vi "子VI-查看某框.vi"(0 "输入框号（默认值0为整张图）":dbl format="%#_13g", 1 "框组":T3(array[cluster]), 2 "判定为筋条的长宽比阈值":i32, 3 "临界Z值":i32, 4 "缺陷灰度阈值":dbl caption="值", 5 "临界面积百分比值":dbl, 6 "计入缺陷的面积阈值":i32, 7 "计入缺陷的Z值阈值":i32 caption="值", 8 "?":T2(plugin-control), 9 "部位信息":string[](array[string])=["", "34.500000", "32.500000", "1121", "34", "54.955926", "分层类", "不合格", ""], 10 "图像Y向分辨率（mm/像素）":dbl, 11 "图像X向分辨率（mm/像素）":dbl) -> (27 "全部检测结果":string[][](table))   [LabVIEW 2018]
uses:
  <vilib>/vision/NI_Vision_Development_Module.lvlib
panel:
  out "测量结果":dbl[][](array[numeric])
  out "中心Y":dbl
  out "中心X":dbl
  in  "返回主界面":bool caption="辅助定性分析"
  in  "Tab Control":T1
  out "?":T2(plugin-control)
  out "Threshold Image":T2(plugin-control)
  out "分层缺陷个数":i32
  out "合格？ 弥散类":string="fencengThreshold"
  out "合格？分层类":string="fencengThreshold"
  out "?":string
  out "面积 (pixels)":i32
  in  "格式字符串 2":string="%f"
  in  "分隔符（'\\'代码显示）":string="\t"
  out "分层测量结果":dbl[][](array[numeric])
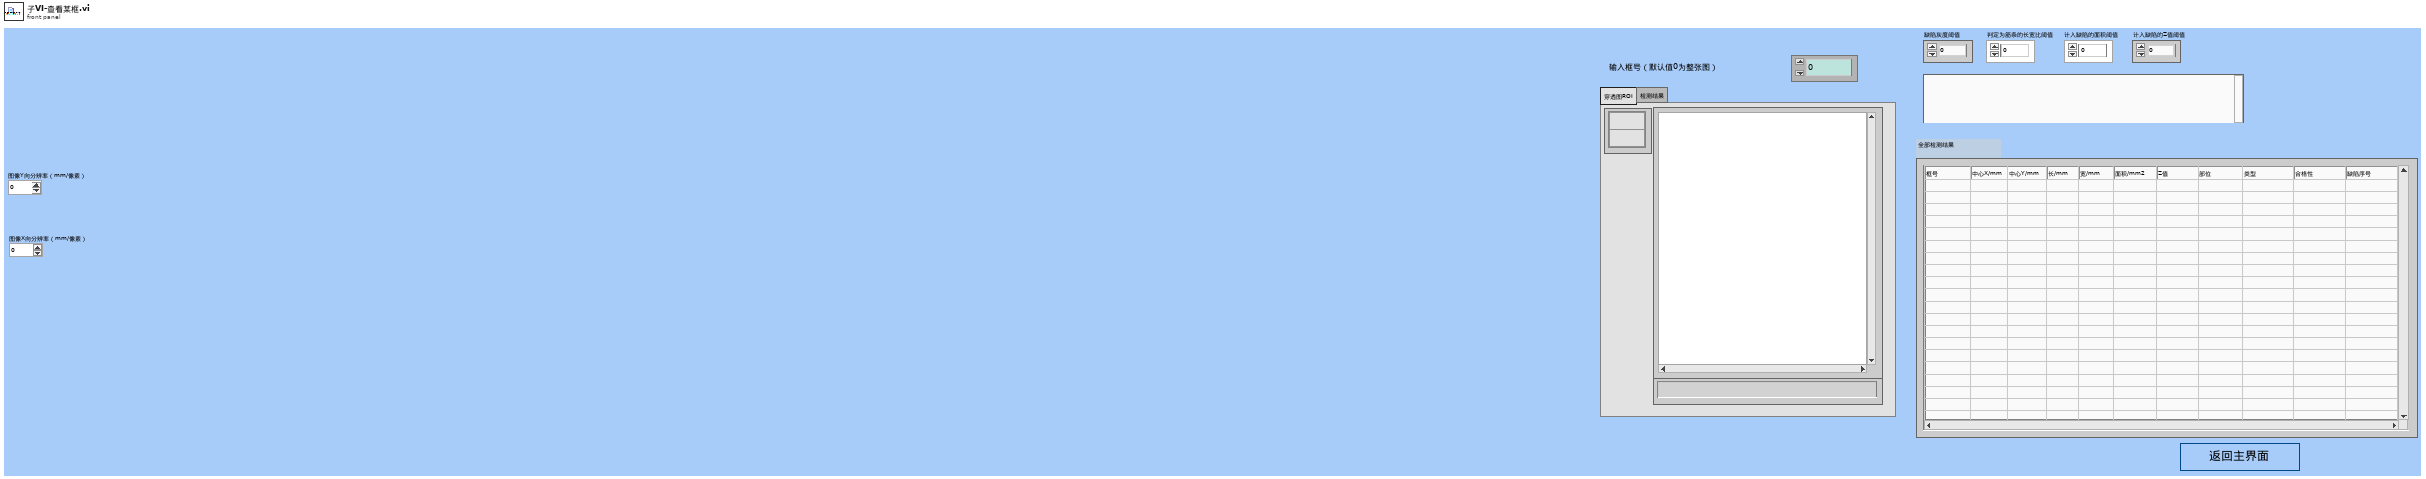
[diagram p1: front panel]
types:
  T1 = typedef "控件2.ctl" = enum32{"穿透图ROI", "检测结果"}
  T2 = typedef "IMAQ Image.ctl" = refnum<image>
  T3 = cluster{"Global Rectangle":i32[], "Contours":cluster{"Contour Type":u32, "ROI Type":u32, "Points":i32[]}[]}[]
  T4 = cluster{"Desired Font (Application)":enum16{"User-specified Font", "Application Font", "System Font", "Dialog Font"}, "[User-specified Font]":cluster{"Font Name":string, "Size":i16, "Strikeout?":bool, "Italic?":bool, "Underline?":bool, "Outline?":bool, "Shadow?":bool, "Bold?":bool, "Rotation Angle":dbl}, "Horizontal Alignment":i16, "Vertical Alignment":i16}
  T5 = cluster{"Zoom Tool":bool, "Selection Tool":bool, "Pan Tool":bool, "Point Tool":bool, "Line Tool":bool, "Rectangle Tool":bool, "Rotated Rectangle Tool":bool, "Polyline Tool":bool, "Polygon Tool":bool, "Freehand Tool":bool, "Closed Freehand Tool":bool, "Ellipse Tool":bool, "Annulus Tool":bool}
  T6 = typedef "Image Type" = u32
  T7 = cluster{"Global Rectangle":i32[], "Contours":cluster{"Contour Type":u32, "ROI Type":u32, "Points":i32[]}[]}
  T8 = cluster{"histogram":u32[], "Minimal Value":sgl, "Maximal Value":sgl, "Starting Value":sgl, "Interval Width":sgl, "Mean Value":sgl, "Standard  Variation":sgl, "Area (pixels)":i32}
  T9 = typedef "Particle Parameters" = i32
  T10 = cluster{"Area":dbl, "Number of Holes":dbl, "Bounding Rect":cluster{"Left":dbl, "Top":dbl, "Right":dbl, "Bottom":dbl}, "Center of Mass":cluster{"X":dbl, "Y":dbl}, "Orientation":dbl, "Dimensions":cluster{"Width":dbl, "Height":dbl}}[]
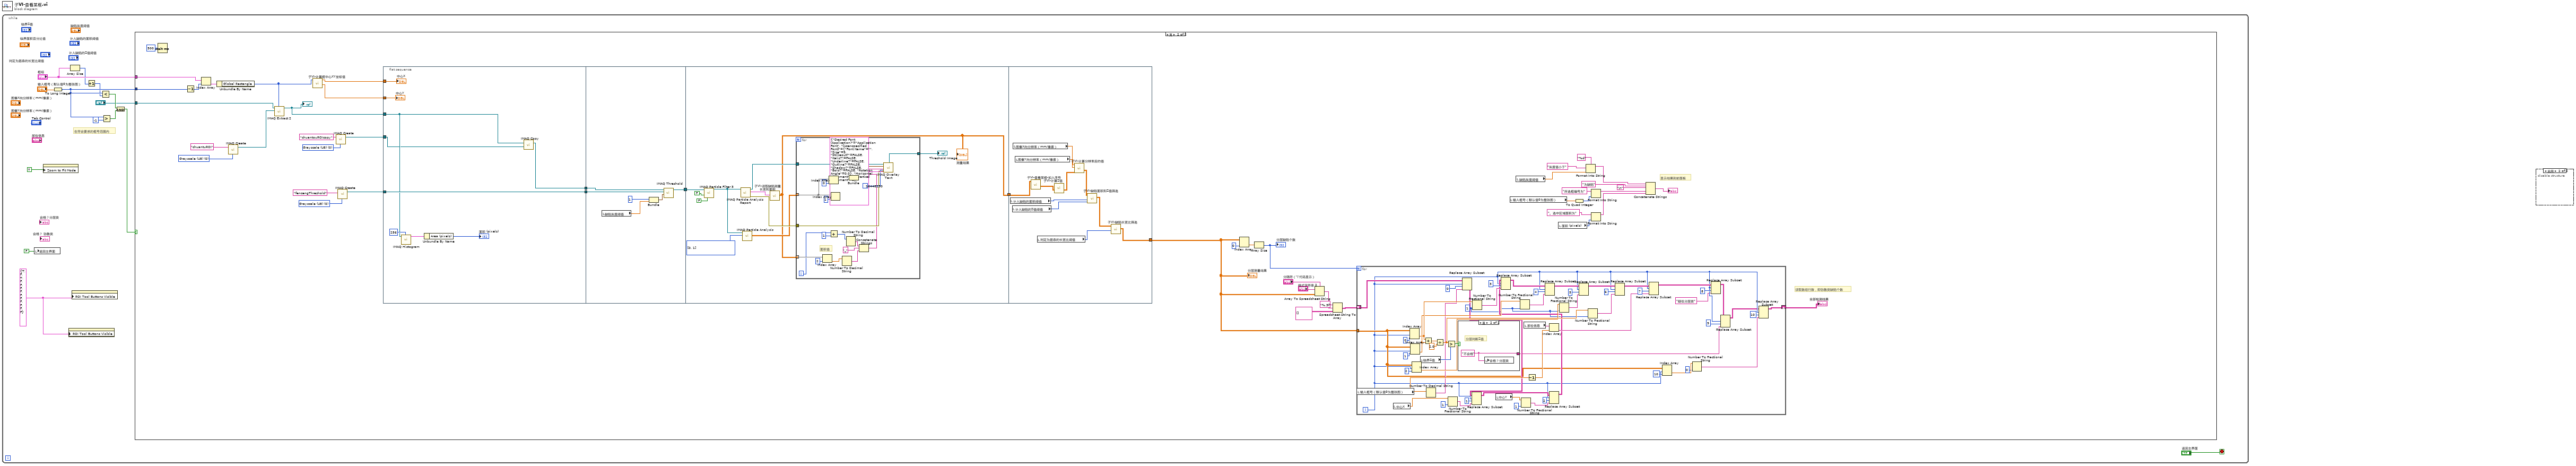
[diagram p0: block diagram]
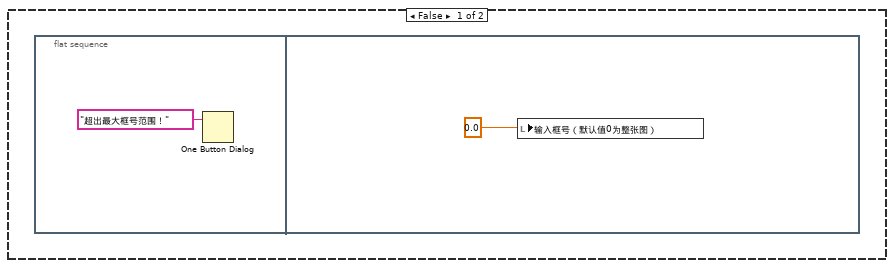
[diagram p2: hidden frame]
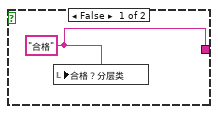
[diagram p3: hidden frame]
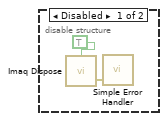
[diagram p4: hidden frame]
diagram:
  n1 = while {
    stop <- "返回主界面" stop-if-true
    w4 = T5 {"Zoom Tool"=TRUE, "Selection Tool"=FALSE, "Pan Tool"=TRUE, "Point Tool"=FALSE, "Line Tool"=FALSE, "Rectangle Tool"=FALSE, "Rotated Rectangle Tool"=FALSE, "Polyline Tool"=FALSE, "Polygon Tool"=FALSE, "Freehand Tool"=FALSE, "Closed Freehand Tool"=FALSE, "Ellipse Tool"=FALSE, "Annulus Tool"=FALSE} ("ROI Tool Buttons Visible:All Elements")
    # "在符合要求的框号范围内"
    n2 = local write "返回主界面"(FALSE ("stop")) -> ()
    n3 = property class="ImageControl"("Zoom to Fit Mode"=TRUE) -> ()  [unwired: 2 in, 2 out]
    n4 = To Long Integer(number="输入框号（默认值0为整张图）") -> (32bit integer=w6:i32)
    n5 = property class="ImageControl"("ROI Tool Buttons Visible"=w4) -> ()  [unwired: 2 in, 2 out]
    n6 = Array Size(array="框组") -> (size(s)=w3:i32)
    n7 = property class="ImageControl"("ROI Tool Buttons Visible"=w4) -> ()  [unwired: 2 in, 2 out]
    n8 = Increment(x=w3) -> (x+1=w2:i32)
    n9 = Less?(x=w6, y=w2) -> (x < y?=w8:bool)
    n10 = Greater?(x=w6, y=-1) -> (0:w7:bool)
    n11 = And(x=w8, y=w7) -> (x .and. y?=w9:bool)
    n12 = case shown="真" w9 {
      tunnel: "框组" -> [_ w29]
      tunnel: w6 -> [_ w28]
      tunnel: "?" -> [_ w20]
      frame False {
        n13 = flat-sequence {
          frame #0 {
            n14 = One Button Dialog(message="超出最大框号范围！" ("消息")) -> ()  [unwired: 1 in, 1 out]
          }
          frame #1 {
            n15 = local write "输入框号（默认值0为整张图）"(0.0 ("框号")) -> ()
          }
        }
      }
      frame True {
        w43 = T6 0 items=["Grayscale (U8)", "Grayscale (I16)", "Grayscale (SGL)", "Complex (CSG)", "RGB (U32)", "HSL (U32)", "RGB (U64)", "Grayscale (U16)"] ("Image Type")
        w55 = T6 0 items=["Grayscale (U8)", "Grayscale (I16)", "Grayscale (SGL)", "Complex (CSG)", "RGB (U32)", "HSL (U32)", "RGB (U64)", "Grayscale (U16)"] ("Image Type")
        w57 = T6 0 items=["Grayscale (U8)", "Grayscale (I16)", "Grayscale (SGL)", "Complex (CSG)", "RGB (U32)", "HSL (U32)", "RGB (U64)", "Grayscale (U16)"] ("Image Type")
        # "显示结果到前面板"
        # "读取数组行数，即弥散类缺陷个数"
        n16 = Wait (ms)(milliseconds to wait=u32 500 ("等待时间（毫秒）")) -> ()  [unwired: 1 out]
        n17 = Decrement(x=w28) -> (x-1=w60:i32)
        n18 = Index Array(array=w29, index=w60) -> (element=w61:T7)
        n19 = Unbundle By Name(w61) -> ("Global Rectangle"=w25:i32[])
        n20 = call "IMAQ Create"("Image Name"="chuantuROI", "Image Type"=w57) -> ("New Image"=w56:T2)  [unwired: 3 in, 1 out]
        n21 = call "IMAQ Extract 2"("Optional Rectangle"=w25, "Image Dst"=w56, "Image Src"=w20) -> ("Image Dst Out"=w19:T2)  [unwired: 7 in, 1 out]
        "?" <- w19
        n22 = call "子VI-计算框中心XY坐标值.vi"("Global Rectangle"=w25) -> ("中心Y"=w23:dbl, "中心X"=w22:dbl)  [unwired: 9 in]
        n23 = call "IMAQ Create"("Image Name"="chuantouROIcopy", "Image Type"=w43) -> ("New Image"=w45:T2)  [unwired: 3 in, 1 out]
        n24 = call "IMAQ Create"("Image Name"="fencengThreshold", "Image Type"=w55) -> ("New Image"=w52:T2)  [unwired: 3 in, 1 out]
        n25 = flat-sequence {
          tunnel: [w133] -> w64
          tunnel: [w128] -> w63
          tunnel: w52 -> [w133]
          tunnel: w19 -> [w129]
          tunnel: w45 -> [w127]
          tunnel: w23 -> [w126]
          tunnel: w22 -> [w125]
          tunnel: w64 -> [w139]
          tunnel: [w134] -> w62
          tunnel: w63 -> [w138]
          tunnel: w62 -> [w147]
          tunnel: [w140] -> w18
          tunnel: [w178] -> w21
          tunnel: w18 -> [w177]
          frame #0 {
            n26 = call "IMAQ Histogram"("Number of Classes"=256, "Image"=w129) -> ("Histogram Report"=w131:T8)  [unwired: 8 in, 1 out]
            n27 = Unbundle By Name(w131) -> ("Area (pixels)"=→"面积 (pixels)":i32)
            n28 = call "IMAQ Copy"("Image Dst"=w127, "Image Src"=w129) -> ("Image Dst Out"=w128:T2)  [unwired: 4 in, 1 out]
            "中心Y" <- w126
            "中心X" <- w125
          }
          frame #1 {
            n29 = local read "缺陷灰度阈值"() -> (w135:dbl)
            n30 = Bundle(1, "缺陷灰度阈值"=w135) -> (w137:cluster{i32, "缺陷灰度阈值":dbl})  [unwired: 1 in]
            n31 = call "IMAQ Threshold"("Range"=w137, "Image Dst"=w139, "Image Src"=w138) -> ("Image Dst Out"=w134:T2)  [unwired: 3 in, 5 out]
          }
          frame #2 {
            w141 = T9[] [0, 1] items=["Center of Mass X", "Center of Mass Y", "First Pixel X", "First Pixel Y", "Bounding Rect Left", "Bounding Rect Top", "Bounding Rect Right", "Bounding Rect Bottom", "Max Feret Diameter Start X", "Max Feret Diameter Start Y", "Max Feret Diameter End X", "Max Feret Diameter End Y", "Max Horiz. Segment Length Left", "Max Horiz. Segment Length Right", "Max Horiz. Segment Length Row", "-", "Bounding Rect Width", "Bounding Rect Height", "Bounding Rect Diagonal", "Perimeter", "Convex Hull Perimeter", "Holes' Perimeter", "Max Feret Diameter", "Equivalent Ellipse Major Axis", "Equivalent Ellipse Minor Axis", "Equivalent Ellipse Minor Axis (Feret)", "Equivalent Rect Long Side", "Equivalent Rect Short Side", "Equivalent Rect Diagonal", "Equivalent Rect Short Side (Feret)", "Average Horiz. Segment Length", "Average Vert. Segment Length", "Hydraulic Radius", "Waddel Disk Diameter", "-", "Area", "Holes' Area", "Particle & Holes' Area", "Convex Hull Area", "Image Area", "-", "Number of Holes", "Number of Horiz. Segments", "Number of Vert. Segments", "-", "Orientation", "Max Feret Diameter Orientation", "-", "% Area/Image Area", "% Area/(Particle & Holes' Area)", "Ratio of Equivalent Ellipse Axes", "Ratio of Equivalent Rect Sides", "-", "Elongation Factor", "Compactness Factor", "Heywood Circularity Factor", "Type Factor", "-", "Sum X", "Sum Y", "Sum XX", "Sum XY", "Sum YY", "Sum XXX", "Sum XXY", "Sum XYY", "Sum YYY", "-", "Moment of Inertia XX", "Moment of Inertia XY", "Moment of Inertia YY", "Moment of Inertia XXX", "Moment of Inertia XXY", "Moment of Inertia XYY", "Moment of Inertia YYY", "Norm. Moment of Inertia XX", "Norm. Moment of Inertia XY", "Norm. Moment of Inertia YY", "Norm. Moment of Inertia XXX", "Norm. Moment of Inertia XXY", "Norm. Moment of Inertia XYY", "Norm. Moment of Inertia YYY", "Hu Moment 1", "Hu Moment 2", "Hu Moment 3", "Hu Moment 4", "Hu Moment 5", "Hu Moment 6", "Hu Moment 7"] ("Pixel Measurements")
            n32 = call "IMAQ Particle Filter 3"("Image Src"=w147, "Keep/Remove Particles (F)"=FALSE, "Reject Border? (F)"=FALSE) -> ("Image Dst Out"=w143:T2)  [unwired: 10 in, 2 out]
            n33 = call "IMAQ Particle Analysis Report"("Image"=w143) -> ("error out"=w144:errorcluster, "Particle Reports (Pixels)"=w148:T10, "Image Out (duplicate)"=w145:T2)  [unwired: 5 in, 3 out]
            n34 = call "IMAQ Particle Analysis"("Pixel Measurements"=w141, "Image"=w143) -> ("Particle Measurements (Pixels)"=w142:dbl[][])  [unwired: 4 in, 5 out]
            n35 = call "子VI-读取缺陷测量长宽和面积.vi"("Particle Reports (Pixels)"=w148) -> ("测量结果"=w140:dbl[][])  [unwired: 10 in]
            "测量结果" <- w140
            n36 = for {
              tunnel: [w163] -> w146
              tunnel: w145 -> [w171]
              tunnel: w142 -> [w168] mode=indexing
              tunnel: w144 -> [w162]
              tunnel: w140 -> [w158] mode=indexing
              i -> [w153]
              # "面积值"
              n37 = Index Array(array=w158, index=2 ("索引")) -> (element=w166:dbl)
              n38 = Index Array(array=w168, index=0 ("索引")) -> (element=w161:dbl)
              n39 = Add(x=w153, y=1) -> (x+y=w151:i32)
              n40 = Index Array(array=w168, index=1 ("索引")) -> (element=w160:dbl)
              n41 = Number To Decimal String(number=w166) -> (decimal integer string=w155:string)  [unwired: 1 in]
              n42 = Number To Decimal String(number=w151) -> (decimal integer string=w157:string)  [unwired: 1 in]
              n43 = Bundle("Numeric"=w161, "Numeric"=w160) -> (w159:cluster{"Numeric":dbl, "Numeric":dbl})  [unwired: 1 in]
              n44 = Concatenate Strings(w157, "_" ("字符串"), w155) -> (w156:string)
              n45 = call "IMAQ Overlay Text"("Text Color (black)"=u32 16448250, "Font, Size & Style"=T4 {"Desired Font (Application)"=enum."Application Font", "[User-specified Font]"={"Font Name"="", "Size"=9, "Strikeout?"=FALSE, "Italic?"=FALSE, "Underline?"=FALSE, "Outline?"=FALSE, "Shadow?"=FALSE, "Bold?"=FALSE, "Rotation Angle"=0.0}, "Horizontal Alignment"=0, "Vertical Alignment"=0}, "error in (no error)"=w162, "String"=w156, "Origin"=w159, "Image"=w171) -> ("Image Out"=w163:T2)  [unwired: 4 in, 1 out]
            }
            "Threshold Image" <- w146
          }
          frame #3 {
            n46 = local read "计入缺陷的面积阈值"() -> (w179:i32)
            n47 = local read "计入缺陷的Z值阈值"() -> (w176:i32)
            n48 = local read "图像X向分辨率（mm/像素）"() -> (w181:dbl)
            n49 = local read "图像Y向分辨率（mm/像素）"() -> (w182:dbl)
            n50 = call "子VI-查看某框-加入序号.vi"("测量结果"=w177) -> ("测量结果 3"=w175:dbl[][])  [unwired: 9 in]
            n51 = local read "判定为筋条的长宽比阈值"() -> (w180:i32)
            n52 = call "子VI-计算Z值.vi"("分层测量结果"=w175) -> ("初始化的数组"=w174:dbl[][])  [unwired: 9 in]
            n53 = call "子VI-计算分辨率后的值.vi"("测量结果"=w174, "图像X向分辨率（mm/像素）"=w181, "图像Y向分辨率（mm/像素）"=w182) -> ("初始化的数组"=w173:dbl[][])  [unwired: 7 in]
            n54 = call "子VI-缺陷面积和Z值筛选.vi"("计入缺陷的Z值阈值"=w176, "计入分层缺陷的面积阈值"=w179, "分层测量结果"=w173) -> ("初始化的数组"=w172:dbl[][])  [unwired: 7 in, 1 out]
            n55 = call "子VI-缺陷长宽比筛选.vi"("判定为筋条的长宽比阈值"=w180, "分层测量结果"=w172) -> ("初始化的数组"=w178:dbl[][])  [unwired: 9 in]
          }
        }
        n56 = Index Array(array=w21, index (col)=0 ("禁用的索引 (列)")) -> (element=w54:dbl[])  [unwired: 1 in]
        n57 = Array Size(array=w54) -> (size(s)=w51:i32)
        "分层缺陷个数" <- w51
        n58 = Array To Spreadsheet String(delimiter (Tab)="分隔符（'\\'代码显示）", array=w21, 3:"格式字符串 2") -> (spreadsheet string=w48:string)
        n59 = Spreadsheet String To Array(format string="%.3f" ("格式字符串"), spreadsheet string=w48, array type (2D Dbl)=string[][] [] ("Array")) -> (array=w46:string[][])  [unwired: 1 in]
        n60 = for {
          N: w51 -> [_]
          tunnel: w21 -> [w74]
          shift-right: [w69] -> w17
          shift-left: w46 -> [w106]
          i -> [w71]
          w79 = i16 1 ("精度(6)")
          n61 = local read "输入框号（默认值0为整张图）"() -> (w113:dbl)
          n62 = local read "中心X"() -> (w90:dbl)
          n63 = Index Array(array=w74, index (row)=w71, index (col)=0 ("禁用的索引 (列)")) -> (element=w98:dbl)
          n64 = Index Array(array=w74, index (row)=w71, index (col)=1 ("禁用的索引 (列)")) -> (element=w97:dbl)
          n65 = Index Array(array=w74, index (row)=w71, index (col)=2 ("索引 (列)")) -> (element=w92:dbl)
          n66 = local read "临界Z值"() -> (w120:i32)
          n67 = Add(x=w98, y=w97) -> (x+y=w121:dbl)
          n68 = Number To Decimal String(number=w113) -> (decimal integer string=w91:string)  [unwired: 1 in]
          n69 = Divide(x=w121, y=2.0) -> (x/y=w95:dbl)
          n70 = Greater?(x=w95, y=w120) -> (0:w122:bool)
          n71 = Number To Fractional String(number=w90, precision (6)=i16 1 ("精度(6)")) -> (F-format string=w85:string)  [unwired: 2 in]
          n72 = case shown="真" w122 {
            tunnel: [w123 w124] -> w66
            frame False {
              w123 = "合格" ("合格？")
              n73 = local write "合格？分层类"(w123) -> ()
            }
            frame True {
              w124 = "不合格" ("合格？")
              # "分层判断Z值"
              n74 = local write "合格？分层类"(w124) -> ()
            }
          }
          n75 = Replace Array Subset(array=w106, new element=w91, index (row)=w71, index (col)=0 ("索引 (列)")) -> (w89:string[][])
          n76 = Replace Array Subset(array=w89, new element=w85, index (row)=w71, index (col)=1 ("禁用的索引 (列)")) -> (w86:string[][])
          n77 = Number To Fractional String(number=w98, precision (6)=w79) -> (F-format string=w105:string)  [unwired: 2 in]
          n78 = local read "中心Y"() -> (w83:dbl)
          n79 = Number To Fractional String(number=w97, precision (6)=w79) -> (F-format string=w104:string)  [unwired: 2 in]
          n80 = Number To Fractional String(number=w83, precision (6)=i16 1 ("精度(6)")) -> (F-format string=w82:string)  [unwired: 2 in]
          n81 = local read "部位信息"() -> (w116:string[])
          n82 = Decrement(x=w113) -> (x-1=w115:dbl)
          n83 = Index Array(array=w116, index=w115) -> (element=w94:string)
          n84 = Replace Array Subset(array=w86, new element=w82, index (row)=w71, index (col)=2 ("索引 (列)")) -> (w84:string[][])
          n85 = Replace Array Subset(array=w84, new element=w105, index (row)=w71, index (col)=3 ("索引 (列)")) -> (w103:string[][])
          n86 = Replace Array Subset(array=w103, new element=w104, index (row)=w71, index (col)=4 ("索引 (列)")) -> (w102:string[][])
          n87 = Number To Fractional String(number=w92, precision (6)=w79) -> (F-format string=w101:string)  [unwired: 2 in]
          n88 = Replace Array Subset(array=w102, new element=w101, index (row)=w71, index (col)=5 ("索引 (列)")) -> (w100:string[][])
          n89 = Number To Fractional String(number=w95, precision (6)=w79) -> (F-format string=w96:string)  [unwired: 2 in]
          n90 = Replace Array Subset(array=w100, new element=w96, index (row)=w71, index (col)=6 ("索引 (列)")) -> (w99:string[][])
          n91 = Replace Array Subset(array=w99, new element=w94, index (row)=w71, index (col)=7 ("索引 (列)")) -> (w78:string[][])
          n92 = Index Array(array=w74, index (row)=w71, index (col)=10 ("索引 (列)")) -> (element=w73:dbl)
          n93 = Number To Fractional String(number=w73, precision (6)=i16 0 ("精度(6)")) -> (F-format string=w65:string)  [unwired: 2 in]
          n94 = Replace Array Subset(array=w78, new element="疑似分层类" ("新元素/子数组"), index (row)=w71, index (col)=8 ("索引 (列)")) -> (w77:string[][])
          n95 = Replace Array Subset(array=w77, new element=w66, index (row)=w71, index (col)=9 ("禁用的索引 (列)")) -> (w70:string[][])
          n96 = Replace Array Subset(array=w70, new element=w65, index (row)=w71, index (col)=10 ("禁用的索引 (列)")) -> (w69:string[][])
        }
        "全部检测结果" <- w17
        n97 = local read "输入框号（默认值0为整张图）"() -> (w37:dbl)
        n98 = local read "缺陷灰度阈值"() -> (w24:dbl)
        n99 = local read "面积 (pixels)"() -> (w40:i32)
        n100 = To Quad Integer(1:w37) -> (0:w38:i64)
        n101 = Format Into String(format string="%d" ("格式字符串"), initial string="灰度值小于" ("初始字符串"), w24) -> (resulting string=w41:string)  [unwired: 1 in, 1 out]
        n102 = Format Into String(initial string="所选框编号为" ("初始字符串"), w38) -> (resulting string=w36:string)  [unwired: 2 in, 1 out]
        n103 = Format Into String(initial string="。选中区域面积为" ("字符串"), w40) -> (resulting string=w42:string)  [unwired: 2 in, 1 out]
        n104 = Concatenate Strings(w41, "为缺陷" ("初始字符串"), "\n", w36, w42) -> (→"?":string)
        "分层测量结果" <- w21
      }
    }
  }
  n105 = disable-structure shown="启用" {
    frame Disabled {
      n106 = call "Imaq Dispose"("All Images? (No)"=TRUE) -> ("error out"=w184:errorcluster)  [unwired: 5 in]
      n107 = call <vilib>:"Simple Error Handler.vi"("error in (no error)"=w184) -> ()  [unwired: 4 in, 5 out]
    }
    frame Enabled {
    }
  }
